vi "Rad to Arcsec.vi"(1 "Radiano":dbl format="%.9g") -> (0 "Arcsec":dbl)   [LabVIEW 2012]
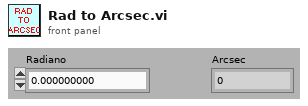
[diagram p1: front panel]
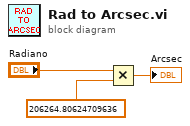
[diagram p0: block diagram]
diagram:
  n1 = Multiply(x="Radiano", y=206264.80624709636) -> (x*y=→"Arcsec":dbl)
